vi "Init.vi"(8 "error in":errorcluster, 11 "CANopen Master in":refnum<class "CANopen Master.lvclass">) -> (0 "error out":errorcluster, 3 "CANopen Master out":refnum<class "CANopen Master.lvclass">)   [LabVIEW 2024, in "CANopen Master.lvlib" / "CANopen Master.lvclass"]
uses:
  CANopen Master.lvclass
  CANopen Master.lvclass/CANopen Master.ctl
  Heartbeat/Heartbeat.lvclass
  SDO Manager/SDO Manager.lvclass
  Network Mangement/Network Mangement.lvclass
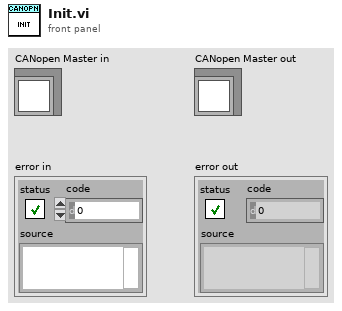
[diagram p1: front panel]
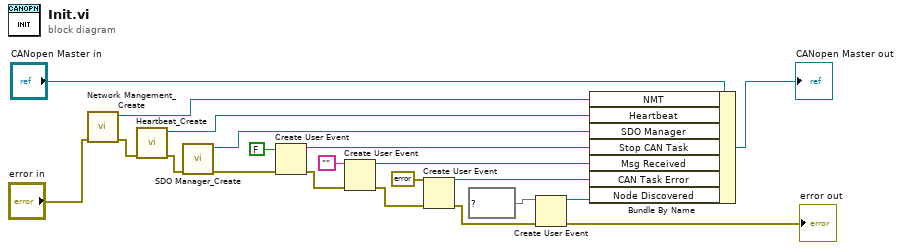
[diagram p0: block diagram]
diagram:
  n1 = call "Network Mangement_Create.vi"("Error In"="error in") -> ("Error Out"=w16:errorcluster, "reference out"=w17:refnum<class "Network Mangement.lvclass">)  [unwired: 9 in]
  n2 = call "Heartbeat_Create.vi"("Error In"=w16) -> ("Error Out"=w18:errorcluster, "reference out"=w20:refnum<class "Heartbeat.lvclass">)  [unwired: 9 in]
  n3 = call "SDO Manager_Create.vi"("Error In"=w18) -> ("Error Out"=w13:errorcluster, "reference out"=w19:refnum<class "SDO Manager.lvclass">)  [unwired: 9 in]
  n4 = Create User Event(user event datatype=FALSE ("Stop CAN Task"), error in=w13) -> (user event=w11:refnum<user-event>, error out=w9:errorcluster)
  n5 = Create User Event(user event datatype="" ("Message Received"), error in=w9) -> (user event=w7:refnum<user-event>, error out=w8:errorcluster)
  n6 = Create User Event(user event datatype=errorcluster {"status"=FALSE, "code"=0, "source"=""} ("Error"), error in=w8) -> (user event=w4:refnum<user-event>, error out=w6:errorcluster)
  n7 = Create User Event(user event datatype=map{u8, u8} {} ("Nodes"), error in=w6) -> (user event=w2:refnum<user-event>, error out=→"error out":errorcluster)
  n8 = Bundle By Name(cluster="CANopen Master in", "NMT"=w17, "Heartbeat"=w20, "SDO Manager"=w19, "Stop CAN Task"=w11, "Msg Received"=w7, "CAN Task Error"=w4, "Node Discovered"=w2) -> (→"CANopen Master out":refnum<class "CANopen Master.lvclass">)
